vi "init_DPV.vi"(3 "input_machine_reference.lvclass":refnum<class "machine.lvclass">) -> (0 "output_DPV_parameters":T1, 1 "output_machine_reference.lvclass":refnum<class "machine.lvclass">)   [LabVIEW 2014, in "technique_parameters.lvclass"]
uses:
  technique_parameters.lvclass
  machine_ops/machine.lvclass
panel:
  in  "Exit":bool
  in  "Set":bool
  in  "Sense Range":T2(ring)
  in  "Quiet time":i32=1800000 min=1000 max=1800000
  in  "Pulse Period":dbl=100.0 min=100.0 max=10000.0
  in  "Pulse Width":dbl=50.0 min=50.0 max=50000.0
  in  "Pulse Amplitude":dbl=1e-05 min=1e-05 max=0.5
  in  "Increment Voltage Level":dbl=1e-05 min=1e-05 max=0.2
  in  "End_Voltage_Level":dbl min=-10.0 max=10.0
  in  "Initial Voltage Level":dbl min=-10.0 max=10.0
  # "V"
  # "ms"
  # "ms"
  # "V"
  # "ms"
  # "V"
  # "A"
  # "V"
  # "Default sample width is 1/10 of pulse period..."
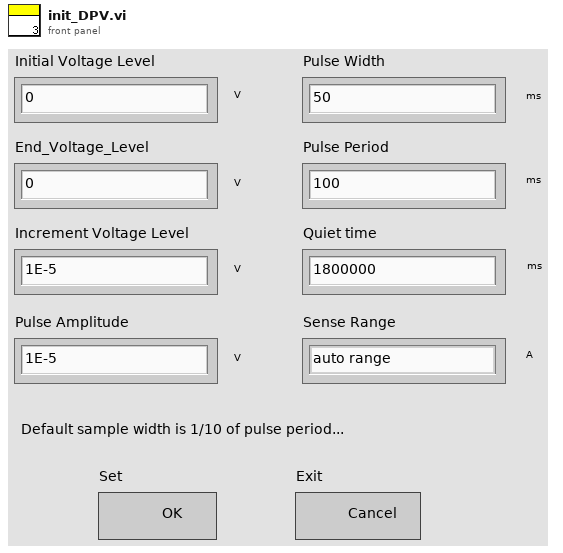
[diagram p1: front panel]
types:
  T1 = cluster{"init_volt":dbl, "end_volt":dbl, "incr_volt":dbl, "pulse_amp":dbl, "pulse_width":dbl, "pulse_period":dbl, "quiet_time":i32, "sense_range":enum16{"auto range", "1E-1", "1E-2", "1E-3", "1E-4", "1E-5", "1E-6", "1E-7", "1E-8", "1E-9"}}
  T2 = enum16{"auto range", "1E-1", "1E-2", "1E-3", "1E-4", "1E-5", "1E-6", "1E-7", "1E-8", "1E-9"}
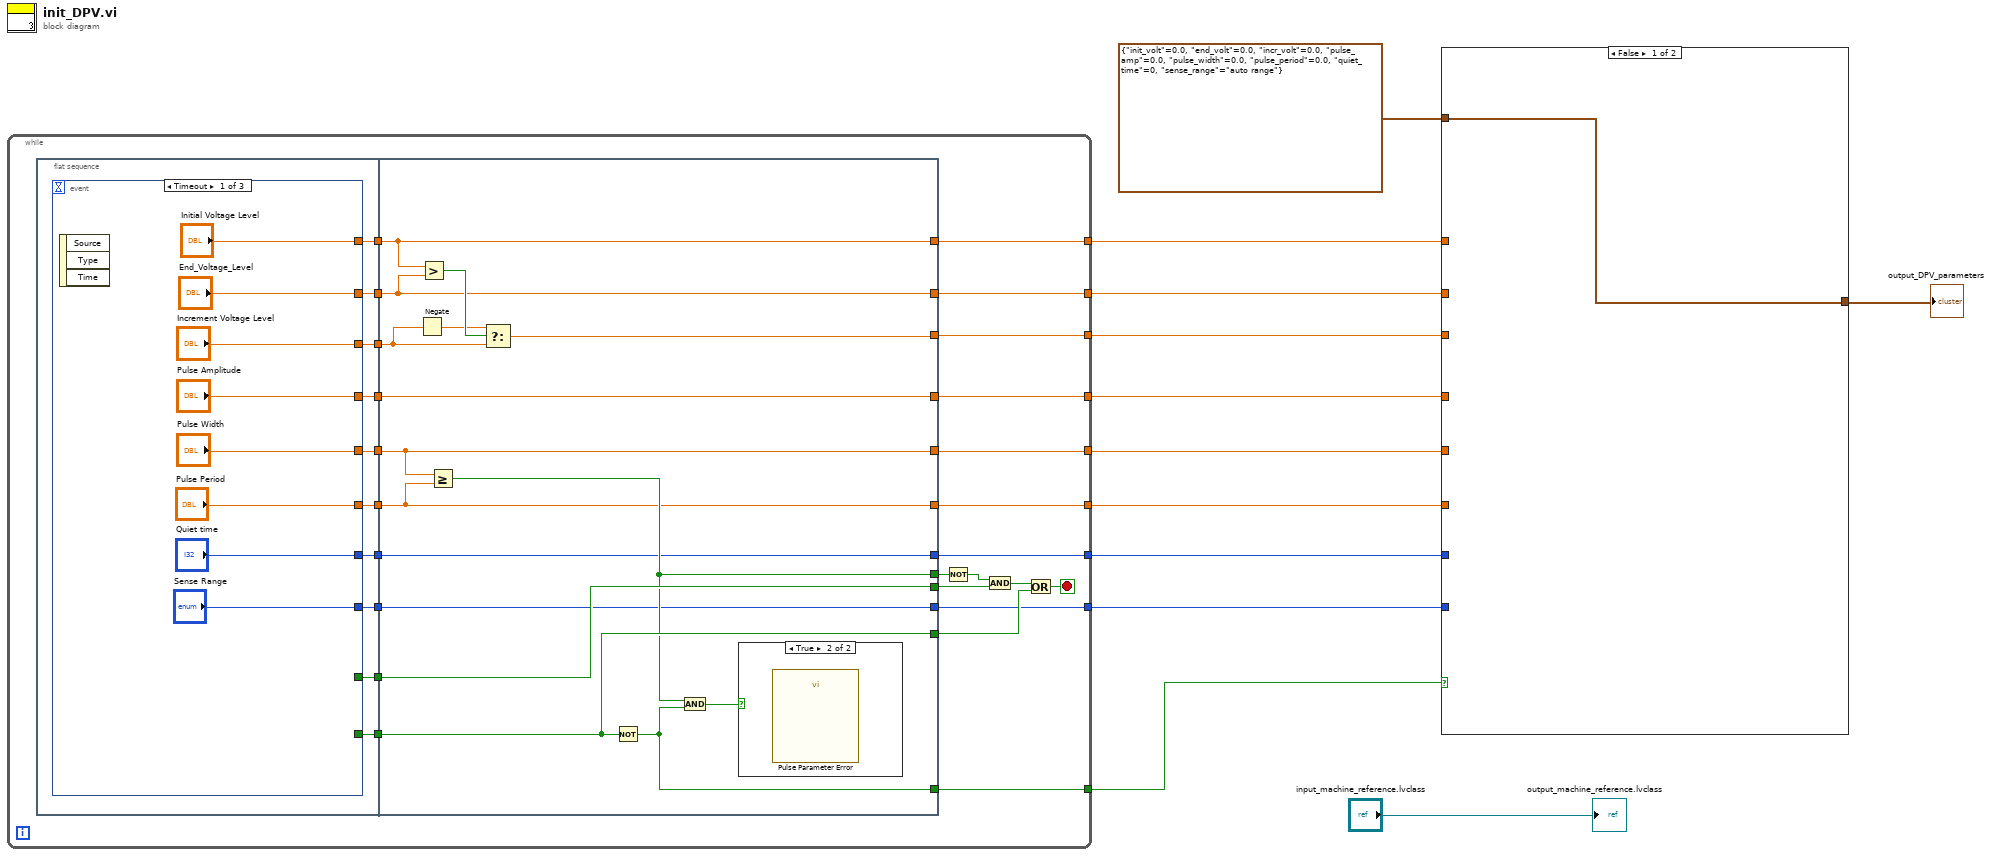
[diagram p0: block diagram]
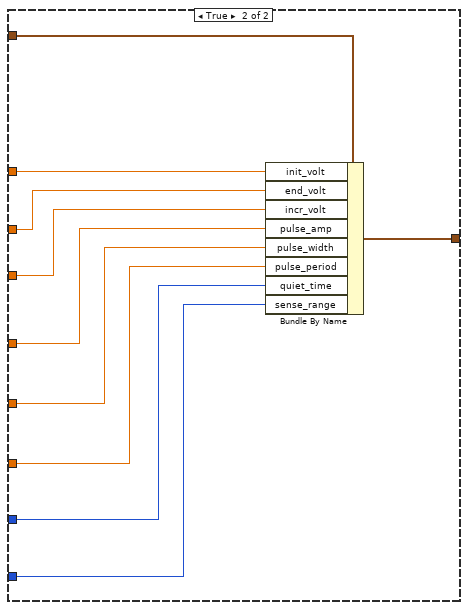
[diagram p2: hidden frame]
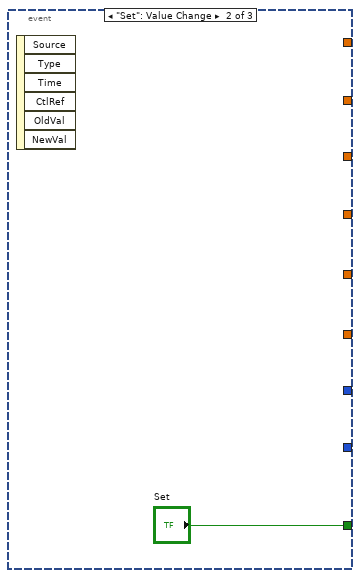
[diagram p3: hidden frame]
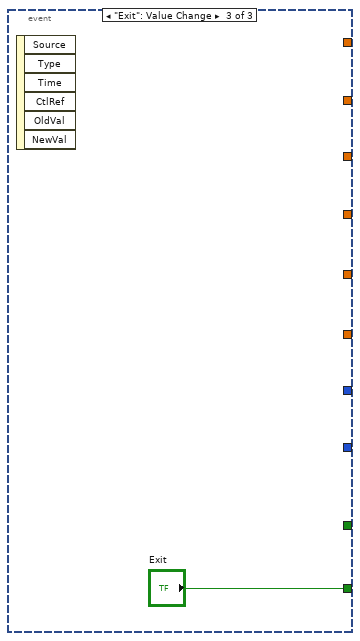
[diagram p4: hidden frame]
diagram:
  n1 = while {
    tunnel: [w21] -> w10
    tunnel: [w20] -> w9
    tunnel: [w19] -> w7
    tunnel: [w18] -> w6
    tunnel: [w17] -> w5
    tunnel: [w16] -> w4
    tunnel: [w15] -> w3
    tunnel: [w14] -> w12
    tunnel: [w13] -> w8
    stop <- w27 stop-if-true
    n2 = flat-sequence {
      tunnel: [w47] -> w37
      tunnel: [w46] -> w36
      tunnel: [w45] -> w35
      tunnel: [w44] -> w34
      tunnel: [w43] -> w33
      tunnel: [w42] -> w32
      tunnel: [w41] -> w31
      tunnel: [w40] -> w30
      tunnel: [w39] -> w29
      tunnel: [w38] -> w28
      tunnel: w37 -> [w66]
      tunnel: w36 -> [w65]
      tunnel: w35 -> [w72]
      tunnel: w34 -> [w64]
      tunnel: w33 -> [w63]
      tunnel: w32 -> [w62]
      tunnel: w31 -> [w61]
      tunnel: w30 -> [w60]
      tunnel: w29 -> [w68]
      tunnel: w28 -> [w69]
      tunnel: [w68] -> w24
      tunnel: [w69] -> w26
      tunnel: [w67] -> w22
      tunnel: [w66] -> w21
      tunnel: [w65] -> w20
      tunnel: [w64] -> w19
      tunnel: [w63] -> w18
      tunnel: [w62] -> w17
      tunnel: [w61] -> w16
      tunnel: [w60] -> w15
      tunnel: [w59] -> w14
      tunnel: [w58] -> w13
      frame #0 {
        n3 = event shown="[0] Timeout" {
          selector: _ -> [_ _ _]
          dyn-events: _ -> [_ _ _]
          timeout: _ -> [_ _ _]
          tunnel: ["Initial Voltage Level" _ _] -> w47
          tunnel: ["End_Voltage_Level" _ _] -> w46
          tunnel: ["Increment Voltage Level" _ _] -> w45
          tunnel: ["Pulse Amplitude" _ _] -> w44
          tunnel: ["Pulse Width" _ _] -> w43
          tunnel: ["Pulse Period" _ _] -> w42
          tunnel: ["Quiet time" _ _] -> w41
          tunnel: ["Sense Range" _ _] -> w40
          tunnel: [_ "Set" _] -> w39
          tunnel: [_ _ "Exit"] -> w38
          event Timeout {
            n4 = event-data() -> ()  [unwired: 1 in, 3 out]
          }
          event "Set": Value Change {
            n5 = event-data() -> ()  [unwired: 1 in, 6 out]
          }
          event "Exit": Value Change {
            n6 = event-data() -> ()  [unwired: 1 in, 6 out]
          }
        }
      }
      frame #1 {
        n7 = Negate(x=w72) -> (-x=w71:dbl)
        n8 = Greater?(x=w66, y=w65) -> (0:w73:bool)
        n9 = Greater Or Equal?(x=w63, y=w62) -> (x >= y?=w67:bool)
        n10 = Select(t=w71, s=w73, f=w72) -> (s? t:f=w58:dbl)
        n11 = Not(x=w69) -> (.not. x?=w59:bool)
        n12 = And(x=w67, y=w59) -> (x .and. y?=w70:bool)
        n13 = case shown="True" w70 {
          frame False {
          }
          frame True {
            n14 = call "Pulse Parameter Error"() -> ()  [unwired: 10 in, 2 out]
          }
        }
      }
    }
    n15 = Not(x=w22) -> (.not. x?=w23:bool)
    n16 = And(x=w23, y=w24) -> (x .and. y?=w25:bool)
    n17 = Or(x=w25, y=w26) -> (x .or. y?=w27:bool)
  }
  n18 = case shown="False" w12 {
    tunnel: T1 {"init_volt"=0.0, "end_volt"=0.0, "incr_volt"=0.0, "pulse_amp"=0.0, "pulse_width"=0.0, "pulse_period"=0.0, "quiet_time"=0, "sense_range"=enum."auto range"} -> [w74 w84]
    tunnel: w10 -> [_ w83]
    tunnel: w9 -> [_ w82]
    tunnel: w8 -> [_ w81]
    tunnel: w7 -> [_ w80]
    tunnel: w6 -> [_ w79]
    tunnel: w5 -> [_ w78]
    tunnel: w4 -> [_ w77]
    tunnel: w3 -> [_ w76]
    tunnel: [w74 w75] -> w2
    frame False {
    }
    frame True {
      n19 = Bundle By Name(cluster=w84, "init_volt"=w83, "end_volt"=w82, "incr_volt"=w81, "pulse_amp"=w80, "pulse_width"=w79, "pulse_period"=w78, "quiet_time"=w77, "sense_range"=w76) -> (w75:T1)
    }
  }
  "output_DPV_parameters" <- w2
  "output_machine_reference.lvclass" <- "input_machine_reference.lvclass"
